vi "PCO_GetActiveLookupTable.vi"(8 "error in (no error)":errorcluster {"code" format="%x"}, 11 "ph":u64) -> (0 "error out":errorcluster {"code" format="%x"}, 1 "wIdentifier":u16, 2 "ErrorMessage":i32 format="%x", 3 "ph out":u64, 5 "wOffset":u16)   [LabVIEW 2019, in "SDK.lvlib" / "ImageSensor.lvlib"]
doc: "<b>Description:</b>\nThis function returns the active lookup table (LUT) in the camera.\n\n<b>Supported camera type:</b>\npco.edge\n\n<b>Descriptor dependency:</b>\nNone"
uses:
  ImageSensor.lvlib
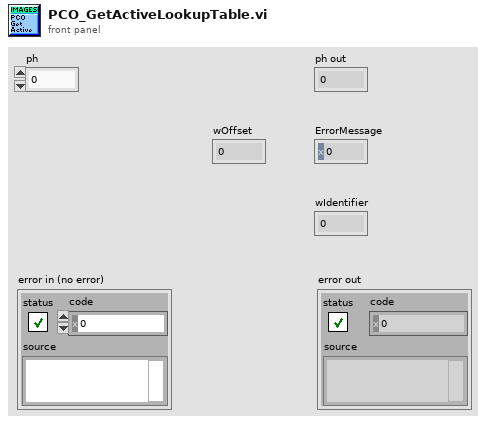
[diagram p1: front panel]
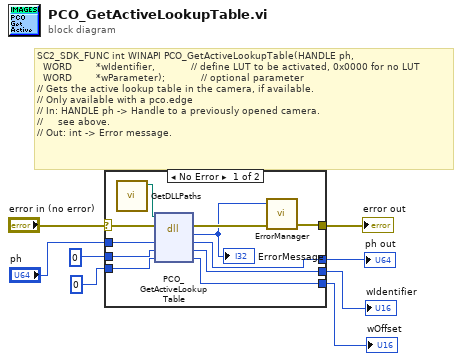
[diagram p0: block diagram]
diagram:
  # "SC2_SDK_FUNC int WINAPI PCO_GetActiveLookupTable(HANDLE ph,\n  WORD        *wIdentifier,            // define LUT to be activated, 0x0000 for no LUT\n  WORD        *wParameter);            // optional parameter\n// Gets the active lookup table in the camera, if available.\n// Only available with a pco.edge\n// In: HANDLE ph -> Handle to a previously opened camera.\n//     see above.\n// Out: int -> Error message."
  n1 = case shown="No Error" "error in (no error)" {
    selector: "error in (no error)" -> [w15 w23]
    tunnel: [w12 w23] -> w8
    tunnel: "ph" -> [w19 w22]
    tunnel: [w18 w22] -> w6
    tunnel: u16 0 ("wIdentifier") -> [w17 w21]
    tunnel: u16 0 ("wParameter") -> [w16 w20]
    tunnel: [w14 w20] -> w2
    tunnel: [w13 w21] -> w1
    frame No Error {
      n2 = call "GetDLLPaths.vi"() -> ("SC2_Cam_Path"=w9:path)  [unwired: 8 in, 3 out]
      n3 = dll-call lib="?" fn="PCO_GetActiveLookupTable"(path in=w9, error in=w15, "ph"=w19, "wIdentifier"=w17, "wOffset"=w16) -> (error out=w11:errorcluster, "return type"=w10:i32, "ph"=w18:u64, "wIdentifier"=w13:u16, "wOffset"=w14:u16)  [unwired: 1 in, 1 out]
      "ErrorMessage" <- w10
      n4 = call "ErrorManager.vi"("error in (no error)"=w11, "error code"=w10) -> ("error out"=w12:errorcluster)  [unwired: 2 in, 1 out]
    }
    frame Error {
    }
  }
  "error out" <- w8
  "ph out" <- w6
  "wOffset" <- w2
  "wIdentifier" <- w1
